vi "Get_KanalInfo.vi"(8 "Error In (No Error)":errorcluster, 11 "VISA Name OZ In (OZ)":refnum<visa-resource-name>="USB0::0x0957::0x179B::MY54313507::INSTR") -> (0 "XORigin":dbl, 1 "YREFerence":dbl, 2 "YORigin":dbl, 3 "YINcrement":dbl, 4 "Error Out":errorcluster, 5 "VISA Name OZ Out":refnum<visa-resource-name>="USB0::0x0957::0x179B::MY54313507::INSTR")   [LabVIEW 2016]
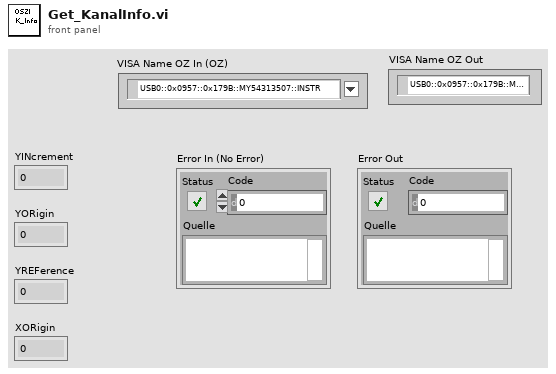
[diagram p1: front panel]
types:
  T1 = cluster{"[0]":refnum<visa-resource-name>, "[1]":refnum<visa-resource-name>, "[2]":refnum<visa-resource-name>, "[3]":refnum<visa-resource-name>, "[4]":refnum<visa-resource-name>, "[5]":refnum<visa-resource-name>, "[6]":refnum<visa-resource-name>, "[7]":refnum<visa-resource-name>, "[8]":refnum<visa-resource-name>}
  T2 = cluster{"[0]":string, "[1]":string, "[2]":string, "[3]":string, "[4]":string, "[5]":string, "[6]":string, "[7]":string, "[8]":string}
  T3 = cluster{"[0]":errorcluster, "[1]":errorcluster, "[2]":errorcluster, "[3]":errorcluster, "[4]":errorcluster, "[5]":errorcluster, "[6]":errorcluster, "[7]":errorcluster, "[8]":errorcluster}
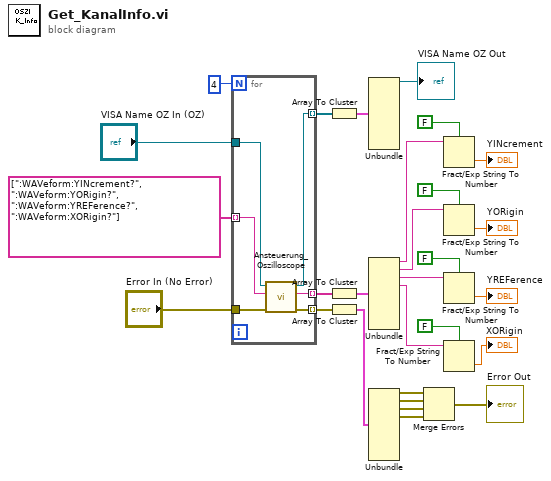
[diagram p0: block diagram]
diagram:
  n1 = for {
    N: 4 -> [_]
    tunnel: [w34] -> w10 mode=indexing
    tunnel: string[] [":WAVeform:YINcrement?", ":WAVeform:YORigin?", ":WAVeform:YREFerence?", ":WAVeform:XORigin?"] -> [w33] mode=indexing
    tunnel: [w32] -> w18 mode=indexing
    tunnel: "Error In (No Error)" -> [w31]
    tunnel: "VISA Name OZ In (OZ)" -> [w30]
    tunnel: [w29] -> w9 mode=indexing
    n2 = call "Ansteuerung_Oszilloscope.vi"("Error_in"=w31, "Eingangs-String"=w33, "VISA Name OZ in(OZ)"=w30) -> ("Error_out"=w34:errorcluster, "Ausgangs-String"=w32:string, "VISA Name OZ out"=w29:refnum<visa-resource-name>)  [unwired: 6 in]
  }
  n3 = Array To Cluster(array=w9) -> (cluster=w8:T1)
  n4 = Array To Cluster(array=w18) -> (cluster=w19:T2)
  n5 = Array To Cluster(array=w10) -> (cluster=w7:T3)
  n6 = Unbundle(w8) -> ("[0]"=→"VISA Name OZ Out":refnum<visa-resource-name>)  [unwired: 8 out]
  n7 = Unbundle(w19) -> ("[0]"=w20:string, "[1]"=w21:string, "[2]"=w23:string, "[3]"=w26:string)  [unwired: 5 out]
  n8 = Unbundle(w7) -> ("[0]"=w6:errorcluster, "[1]"=w5:errorcluster, "[2]"=w4:errorcluster, "[3]"=w3:errorcluster)  [unwired: 5 out]
  n9 = Merge Errors(w6, w5, w4, w3) -> (→"Error Out":errorcluster)
  n10 = Fract/Exp String To Number(use system decimal point (T)=FALSE, string=w20) -> (number=→"YINcrement":dbl)  [unwired: 2 in, 1 out]
  n11 = Fract/Exp String To Number(use system decimal point (T)=FALSE, string=w21) -> (number=→"YORigin":dbl)  [unwired: 2 in, 1 out]
  n12 = Fract/Exp String To Number(use system decimal point (T)=FALSE, string=w23) -> (number=→"YREFerence":dbl)  [unwired: 2 in, 1 out]
  n13 = Fract/Exp String To Number(use system decimal point (T)=FALSE, string=w26) -> (number=→"XORigin":dbl)  [unwired: 2 in, 1 out]
